vi "resetDataPoints.vi"(8 "error in (no error)":errorcluster, 11 "StiffnessCalculator in":refnum<class "StiffnessCalculator.lvclass">) -> (0 "error out":errorcluster, 3 "StiffnessCalculator out":refnum<class "StiffnessCalculator.lvclass">)   [LabVIEW 2015, in "StiffnessCalculator.lvclass"]
uses:
  StiffnessCalculator.lvclass
  StiffnessCalculator.lvclass/StiffnessCalculator.ctl
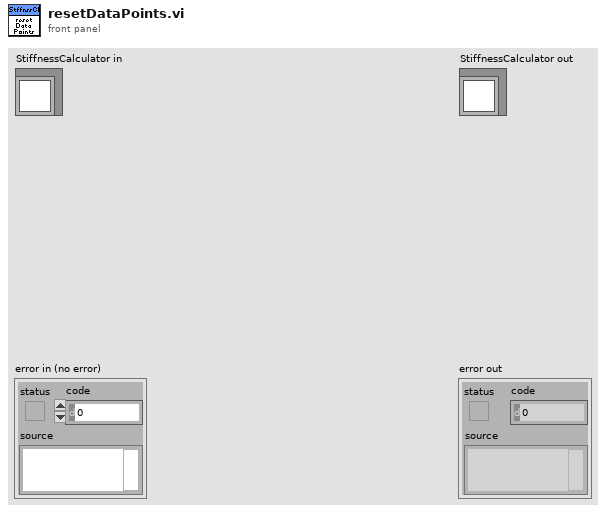
[diagram p1: front panel]
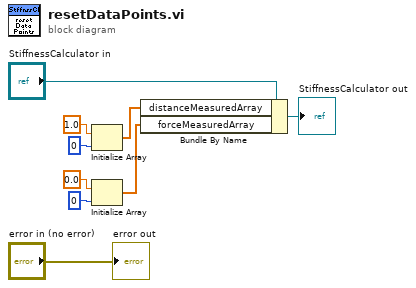
[diagram p0: block diagram]
diagram:
  n1 = Initialize Array(dbl[unit] 1.0 ("Distance Measured"), 0 ("dimension size")) -> (w6:dbl[unit][])
  n2 = Initialize Array(dbl[unit] 0.0 ("Force Measured"), 0 ("dimension size")) -> (w1:dbl[unit][])
  n3 = Bundle By Name(cluster="StiffnessCalculator in", "distanceMeasuredArray"=w6, "forceMeasuredArray"=w1) -> (→"StiffnessCalculator out":refnum<class "StiffnessCalculator.lvclass">)
  "error out" <- "error in (no error)"
